vi "BRig_arrTrig_Cue2Audio_R.vi"() -> (2 "output_Cue2Audio_R":i32)   [LabVIEW 2014]
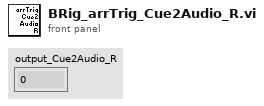
[diagram p1: front panel]
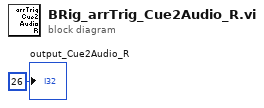
[diagram p0: block diagram]
diagram:
  "output_Cue2Audio_R" <- 26
